vi "LvHostsEdit4cRIO_SUB_LoginInfo_Global.vi"() -> ()   [LabVIEW 2014]
panel:
  in  "password":string
  in  "userID":string
  in  "host":string
  # "IP or hostname"
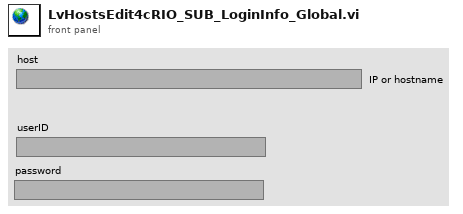
[diagram p1: front panel]
diagram:
